vi "GVmotor_eval_current_turn.vi"(6 "move_pre_sign":i32, 8 "error in":errorcluster, 9 "backlash_corr":bool=TRUE caption="Backlash Correction", 10 "status_code":i32, 11 "VISA in":refnum<visa-resource-name>) -> (0 "error out":errorcluster, 1 "step_curr":i32, 2 "turn_curr":dbl, 3 "VISA out":refnum<visa-resource-name>)   [LabVIEW 2019]
panel:
  out "not_moving":bool
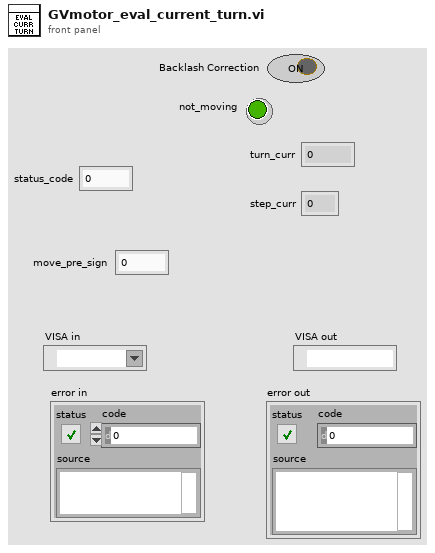
[diagram p1: front panel]
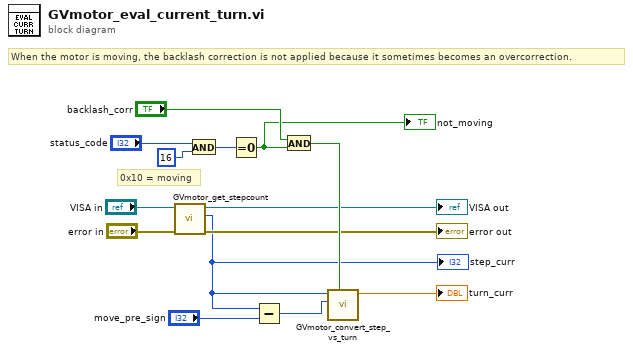
[diagram p0: block diagram]
diagram:
  # "When the motor is moving, the backlash correction is not applied because it sometimes becomes an overcorrection."
  # "0x10 = moving"
  n1 = call "GVmotor_get_stepcount.vi"("error in"="error in", "VISA in"="VISA in") -> ("error out"=→"error out":errorcluster, "Step"=w1:i32, "VISA out"=→"VISA out":refnum<visa-resource-name>)  [unwired: 7 in]
  "step_curr" <- w1
  n2 = And(x="status_code", y=16) -> (x .and. y?=w11:i32)
  n3 = Equal To 0?(x=w11) -> (x = 0?=w10:bool)
  "not_moving" <- w10
  n4 = Subtract(x=w1, y="move_pre_sign") -> (x-y=w3:i32)
  n5 = And(x="backlash_corr", y=w10) -> (x .and. y?=w9:bool)
  n6 = call "GVmotor_convert_step_vs_turn.vi"("backlash_corr"=w9, "step_in_pre"=w3, "step_in"=w1) -> ("turn_out"=→"turn_curr":dbl)  [unwired: 4 in, 4 out]
